vi "AO stage.vi"() -> ()   [LabVIEW 2020]
uses:
  <vilib>/DAQmx/write.llb/DAQmx Write (Analog Wfm 1Chan NSamp).vi
  <vilib>/DAQmx/create/channels.llb/DAQmx Create Channel (AO-Voltage-Basic).vi
  <vilib>/DAQmx/configure/timing.llb/DAQmx Timing (Sample Clock).vi
  <vilib>/DAQmx/miscellaneous.llb/DAQmx Fill In Error Info.vi
panel:
  in  "Stop":bool
  out "Number of slices":dbl
  in  "End position (mm)":dbl
  out "x = y?":bool
  out "last value inside of loop":dbl
  out "Waveform Graph":waveform(dbl)(graph)
  out "last value outside of loop":dbl
  out "Total Z thickness (mm)":dbl
  in  "Z slice width (mm)":dbl
  in  "Start position(mm)":dbl
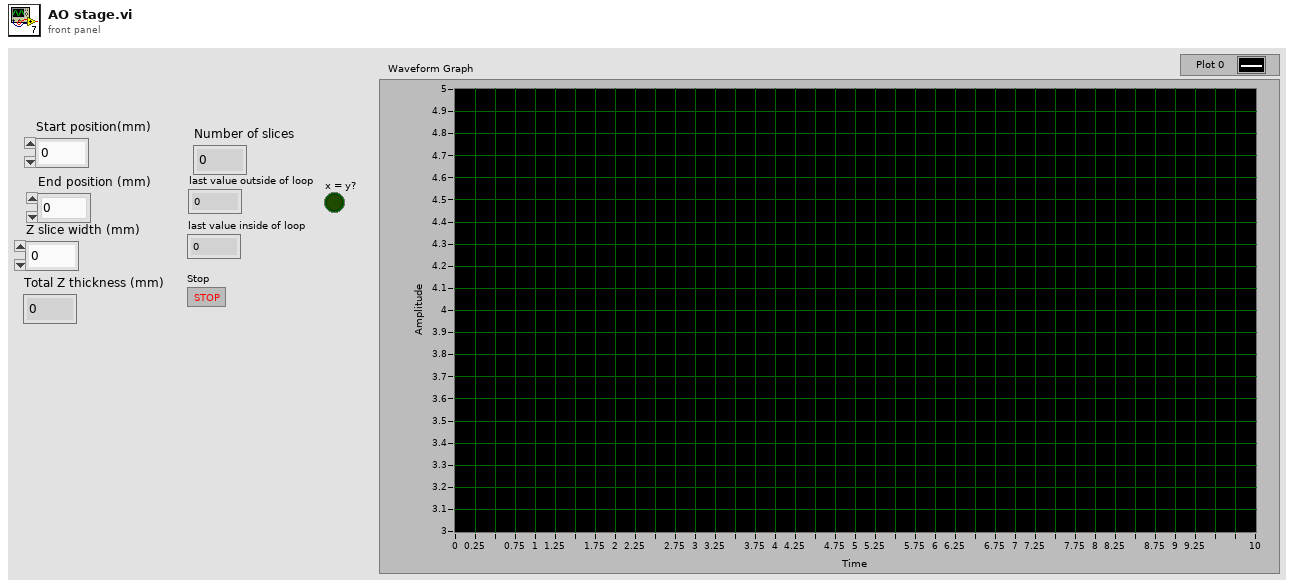
[diagram p1: front panel]
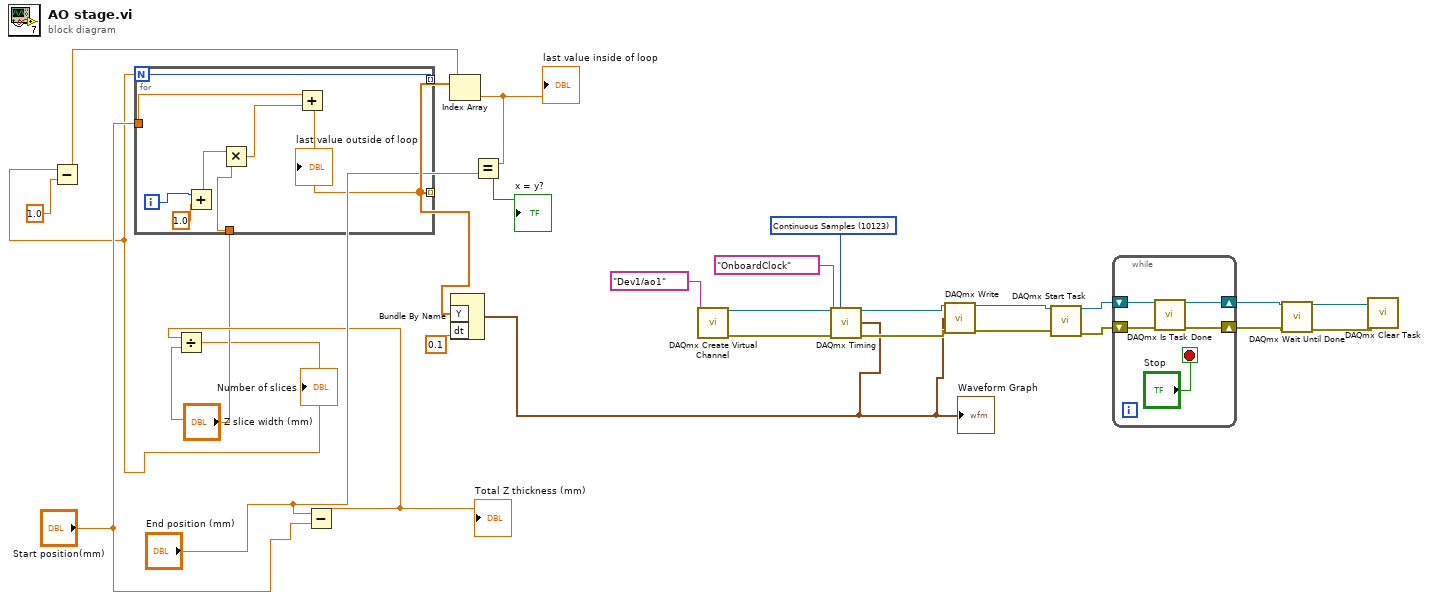
[diagram p0: block diagram]
diagram:
  w18 = 10123 items=["Finite Samples"=10178, "Continuous Samples"=10123, "Hardware Timed Single Point"=12522] ("sample mode")
  n1 = Subtract(x="End position (mm)", y="Start position(mm)") -> (x-y=w8:dbl)
  "Total Z thickness (mm)" <- w8
  n2 = Divide(x=w8, y="Z slice width (mm)") -> (x/y=w6:dbl)
  "Number of slices" <- w6
  n3 = Subtract(x=w6, y=1.0) -> (x-y=w12:dbl)
  n4 = for {
    N: w6 -> [w28]
    tunnel: "Start position(mm)" -> [w35]
    tunnel: "Z slice width (mm)" -> [w34]
    tunnel: [w32] -> w16 mode=indexing
    tunnel: [w28] -> _ mode=indexing
    i -> [w30]
    n5 = Add(x=w30, y=1.0) -> (x+y=w29:dbl)
    n6 = Multiply(x=w29, y=w34) -> (x*y=w33:dbl)
    n7 = Add(x=w35, y=w33) -> (x+y=w32:dbl)
    "last value outside of loop" <- w32
  }
  n8 = Index Array(array=w16, index=w12) -> (element=w14:dbl)
  "last value inside of loop" <- w14
  n9 = Bundle By Name("Y"=w16, "dt"=0.1 ("frequency")) -> (w11:waveform(dbl))  [unwired: 1 in]
  "Waveform Graph" <- w11
  n10 = Equal?(x=w14, y="End position (mm)") -> (x = y?=→"x = y?":bool)
  n11 = call-poly <vilib>:"DAQmx Create Virtual Channel.vi"("physical channels"=tag "Dev1/ao1") -> ("task out"=w27:refnum<k21>, "error out"=w26:errorcluster)  [unwired: 13 in]
  n12 = call-poly <vilib>:"DAQmx Timing.vi"("task/channels in"=w27, "sample mode"=w18, "rate"=w11, "source"=tag "OnboardClock", "error in"=w26) -> ("task out"=w24:refnum<k21>, "error out"=w23:errorcluster)  [unwired: 9 in]
  n13 = call-poly <vilib>:"DAQmx Write.vi"("task/channels in"=w24, "data"=w11, "error in"=w23) -> ("task out"=w22:refnum<k21>, "error out"=w21:errorcluster)  [unwired: 10 in, 1 out]
  n14 = call <vilib>:"DAQmx Start Task.vi"("task/channels in"=w22, "error in"=w21) -> ("task out"=w4:refnum<k21>, "error out"=w3:errorcluster)  [unwired: 12 in]
  n15 = while {
    shift-right: [w38] -> w2
    shift-left: w4 -> [w40]
    shift-right: [w37] -> w1
    shift-left: w3 -> [w39]
    stop <- "Stop" stop-if-true
    n16 = call <vilib>:"DAQmx Is Task Done.vi"("task/channels in"=w40, "error in"=w39) -> ("task out"=w38:refnum<k21>, "error out"=w37:errorcluster)  [unwired: 11 in, 1 out]
  }
  n17 = call <vilib>:"DAQmx Wait Until Done.vi"("task/channels in"=w2, "error in"=w1) -> ("task out"=w20:refnum<k21>, "error out"=w19:errorcluster)  [unwired: 12 in]
  n18 = call <vilib>:"DAQmx Clear Task.vi"("task in"=w20, "error in"=w19) -> ()  [unwired: 13 in, 1 out]
